vi "Insert File into List.vi"(8 "error in (no error)":errorcluster, 9 "Insert in front":bool=TRUE, 10 "File":path, 11 "Plot in":refnum<class "Plot.lvclass">) -> (0 "error out":errorcluster, 3 "Plot out":refnum<class "Plot.lvclass">)   [LabVIEW 2019, in "Plot.lvclass"]
uses:
  Plot.lvclass
  Plot.lvclass/Plot.ctl
  Read Files.vi
  Read File history depth.vi
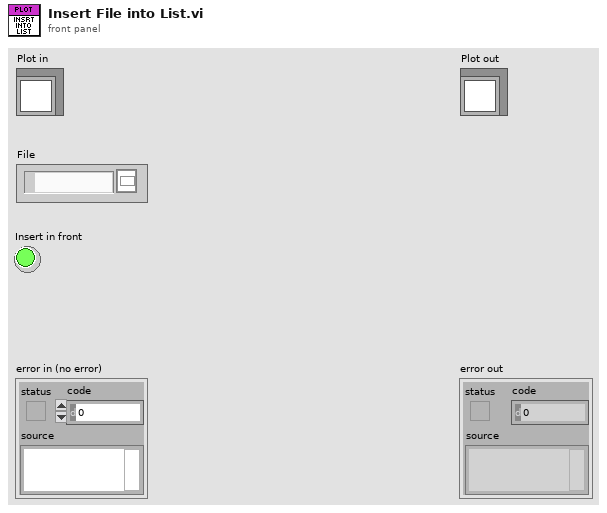
[diagram p1: front panel]
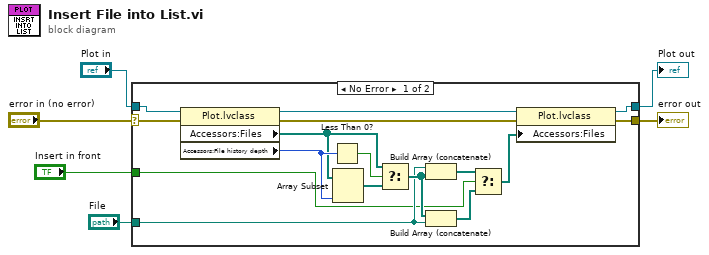
[diagram p0: block diagram]
diagram:
  n1 = case shown="No Error" "error in (no error)" {
    selector: "error in (no error)" -> [w8 w24]
    tunnel: [w7 w24] -> w5
    tunnel: [w9 w23] -> w3
    tunnel: "Plot in" -> [w10 w23]
    tunnel: "File" -> [w12 _]
    tunnel: "Insert in front" -> [w11 _]
    frame No Error {
      n2 = property class="Plot.lvclass"(reference=w10, error in=w8) -> (reference out=w22:refnum<class "Plot.lvclass">, error out=w13:errorcluster, "Accessors:Files"=w19:path[], "Accessors:File history depth"=w21:i32)
      n3 = Less Than 0?(x=w21) -> (x < 0?=w20:bool)
      n4 = Array Subset(array=w19, length=w21) -> (w18:path[])  [unwired: 1 in]
      n5 = Select(t=w19, s=w20, f=w18) -> (s? t:f=w15:path[])
      n6 = Build Array (concatenate)(w12, w15) -> (w17:path[])
      n7 = Build Array (concatenate)(w15, w12) -> (w16:path[])
      n8 = Select(t=w17, s=w11, f=w16) -> (s? t:f=w14:path[])
      n9 = property class="Plot.lvclass"(reference=w22, error in=w13, "Accessors:Files"=w14) -> (reference out=w9:refnum<class "Plot.lvclass">, error out=w7:errorcluster)
    }
    frame Error {
    }
  }
  "error out" <- w5
  "Plot out" <- w3
